vi "Delivery_boa.vi"() -> ()   [LabVIEW 2016]
uses:
  <vilib>/NXT/Subs/LVHSConnector.ctl
  <vilib>/NXT/LegoClasses/BrickReference/BrickReference.lvclass
  caracteristicas.ctl
  <vilib>/NXT/Subs/ColorSensorColors.ctl
  parametros.ctl
  <vilib>/NXT/Block Support/NXT_InputPort.ctl
  <vilib>/NXT/Block Support/NXT_OutputPort.ctl
  <vilib>/NXT/NXTIO Xnodes/NXTIONodeSubVIs/NXTMoveMotors.vi
  <vilib>/NXT/Dual Mode Library/Waits/Wait_Num.vi
  <vilib>/NXT/NXTIO Xnodes/NXTIONodeSubVIs/NXTStopMotors.vi
  <vilib>/NXT/NXTIO Xnodes/AddressXNode/NXTIOAddress.xnode
  <vilib>/NXT/NXTIO Xnodes/NXTIOXNode/NXTIO.xnode
panel:
  in  "Parâmetros Iniciais":T1={"Gyro Port"=0, "Sensor - Left"=3, "Sensor - Right"=2, "     Color \nSensor Port"=1, "Kp Front"=0.6, "Motor speed"=-15, "Distance to street"=20.0, "Motor speed turns"=16, "Kp Curvas"=0.3} {"Kp Front" format="%.3f"; "Color \nSensor Port" items=["Port 1", "Port 2", "Port 3", "Port 4"]; "Sensor - Right" items=["Port 1", "Port 2", "Port 3", "Port 4"]; "Sensor - Left" items=["Port 1", "Port 2", "Port 3", "Port 4"]; "Gyro Port" items=["Port 1", "Port 2", "Port 3", "Port 4"]}
  in  "Características Iniciais":T3={"Colors and Directions"=[enum."Zero", enum."Zero", enum."Zero", enum."Zero", enum."Zero", enum."Zero"], "Direction"=enum."Zero", "CS"=enum."Street", "Old Color"=enum."White"}
  out "Boolean":bool=TRUE
  in  "NXT/EV3":T5
  # "black"
  # "blue"
  # "green"
  # "yellow"
  # "red"
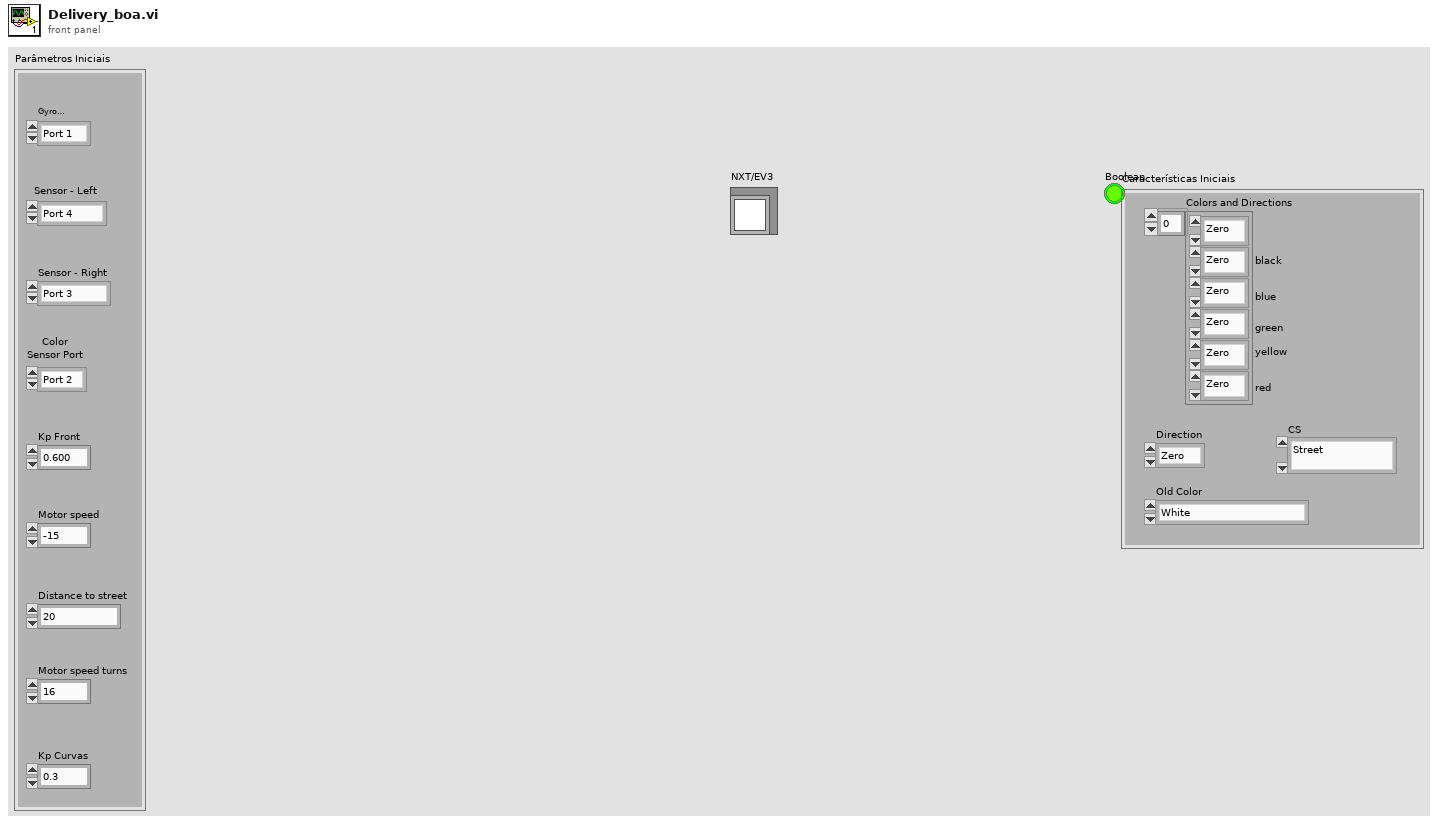
[diagram p1: front panel]
types:
  T1 = typedef "parametros.ctl" = cluster{"Gyro Port":T2, "Sensor - Left":T2, "Sensor - Right":T2, "     Color \nSensor Port":T2, "Kp Front":dbl, "Motor speed":i32, "Distance to street":dbl, "Motor speed turns":i32, "Kp Curvas":dbl}
  T2 = typedef "NXT_InputPort.ctl" = u32
  T3 = typedef "caracteristicas.ctl" = cluster{"Colors and Directions":enum16{"Zero", "Right", "Front", "Left"}[], "Direction":enum16{"Zero", "Right", "Front", "Left"}, "CS":enum16{"Street", "Intersection", "End", "Stop", "Square", "Delivery", "Empty"}, "Old Color":T4}
  T4 = typedef "ColorSensorColors.ctl" = enum16{"No Color", "Black", "Blue", "Green", "Yellow", "Red", "White", "Brown"}
  T5 = typedef "LVHSConnector.ctl" = refnum<class "BrickReference.lvclass">
  T6 = typedef "NXT_OutputPort.ctl" = u8
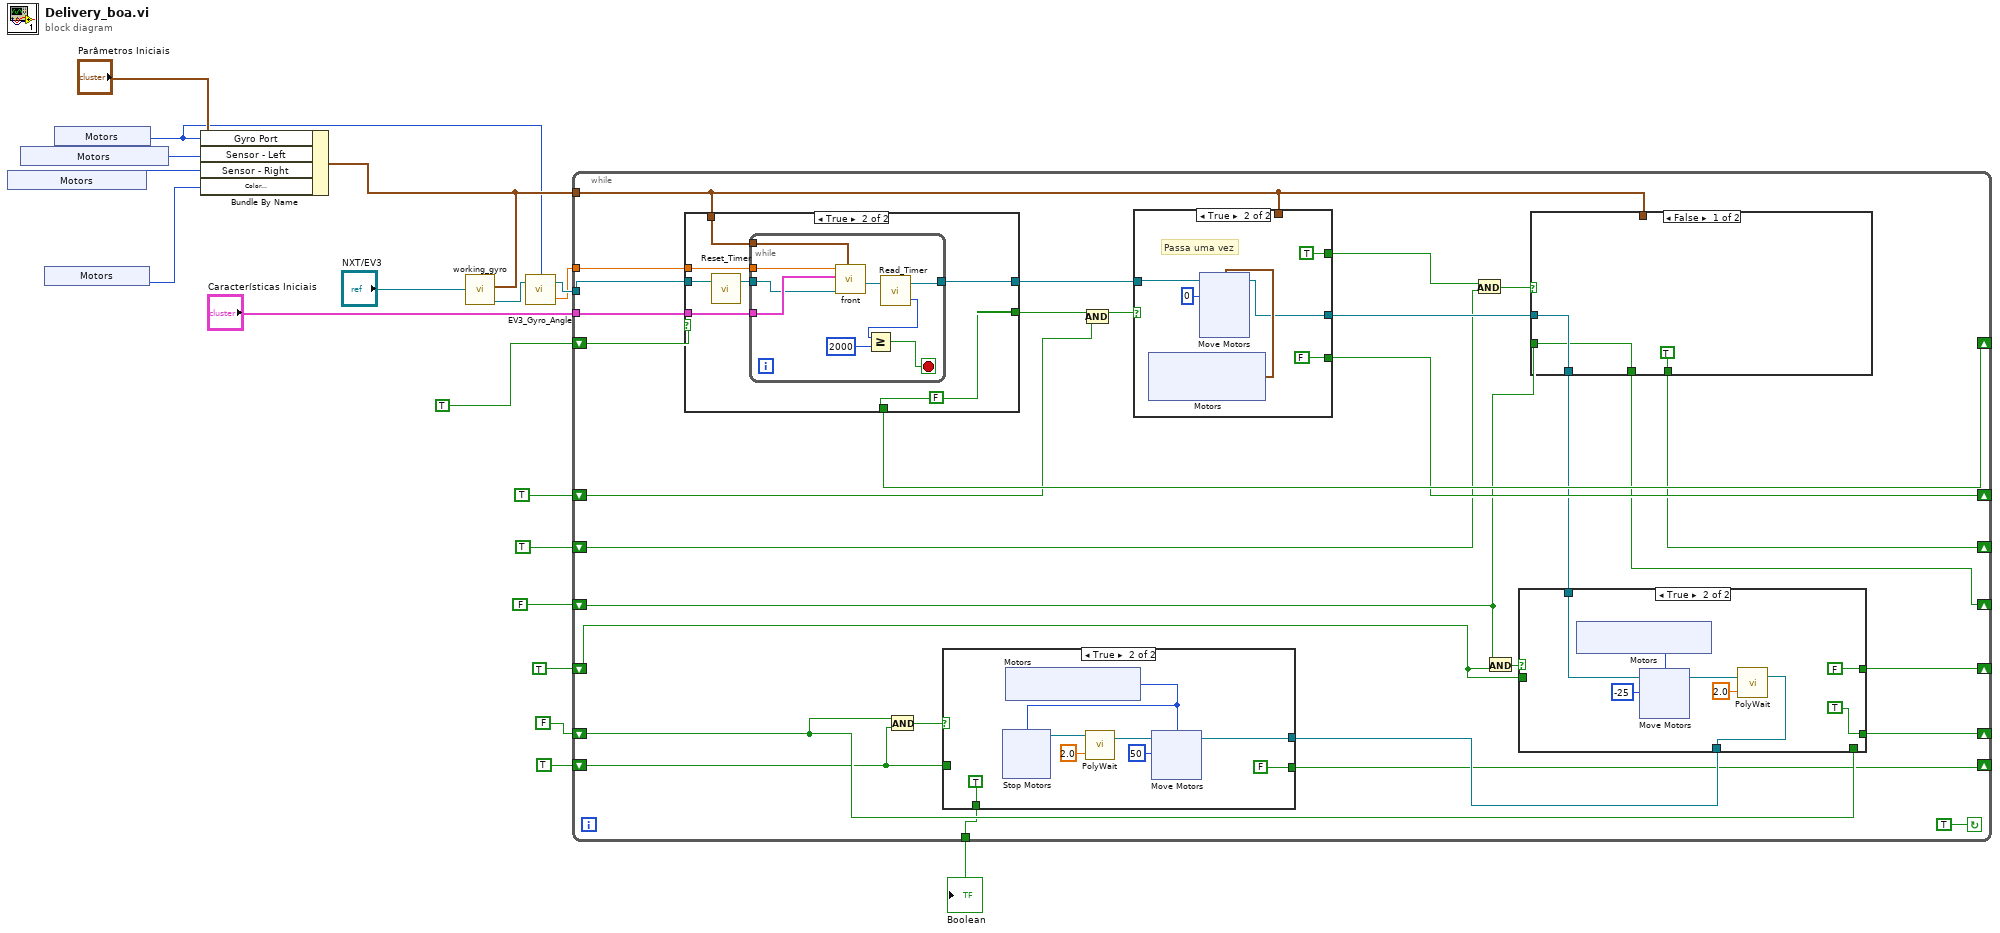
[diagram p0: block diagram]
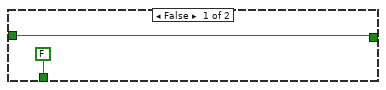
[diagram p2: hidden frame]
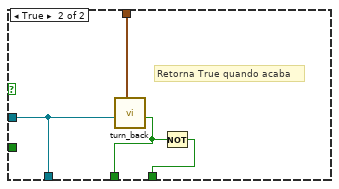
[diagram p4: hidden frame]
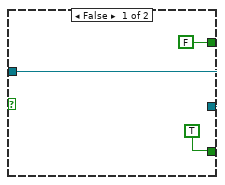
[diagram p5: hidden frame]
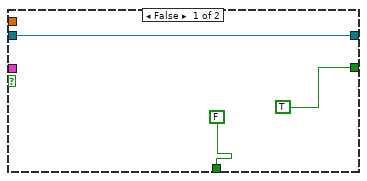
[diagram p6: hidden frame]
diagram:
  n1 = xnode "Motors"() -> ("Sensor"=w8:T2)
  n2 = xnode "Motors"() -> ("Sensor"=w9:T2)
  n3 = xnode "Motors"() -> ("Sensor"=w7:T2)
  n4 = xnode "Motors"() -> ("Sensor"=w1:T2)
  n5 = Bundle By Name(cluster="Parâmetros Iniciais", "Gyro Port"=w1, "Sensor - Left"=w9, "Sensor - Right"=w8, "Color \nSensor Port"=w7) -> (w5:T1)
  n6 = call "working_gyro.vi"("Parâmetros Iniciais"=w5, "NXT/EV3"="NXT/EV3") -> ("NXT/EV3 2"=w3:T5)  [unwired: 9 in]
  n7 = call <vilib>:"EV3_Gyro_Angle.vi"("NXT/EV3"=w3, "Port (Port 1)"=w1) -> ("Degrees"=w2:sgl, "NXT/EV3"=w4:T5)  [unwired: 1 in]
  n8 = while {
    tunnel: w4 -> [w49]
    tunnel: w2 -> [w48]
    shift-right: [w45] -> _
    shift-left: TRUE -> [w47]
    shift-right: [w40] -> _
    shift-left: TRUE -> [w43]
    tunnel: w5 -> [w20]
    shift-right: [w36] -> _
    shift-left: TRUE -> [w38]
    shift-right: [w34] -> _
    shift-left: FALSE -> [w32]
    shift-right: [w31] -> _
    shift-left: TRUE -> [w30]
    shift-right: [w28] -> _
    shift-left: FALSE -> [w26]
    shift-right: [w25] -> _
    shift-left: TRUE -> [w24]
    tunnel: [w23] -> w12
    tunnel: "Características Iniciais" -> [w21]
    stop <- TRUE continue-if-true
    n9 = case shown="True" w47 {
      tunnel: w49 -> [w118 w122]
      tunnel: w48 -> [_ w126]
      tunnel: [TRUE w125] -> w44
      tunnel: [w118 w120] -> w46
      tunnel: [FALSE w125] -> w45
      tunnel: w21 -> [_ w124]
      tunnel: w20 -> [_ w123]
      frame False {
      }
      frame True {
        w125 = FALSE
        n10 = call <vilib>:"Reset_Timer.vi"("NXT/EV3"=w122) -> ("NXT/EV3"=w121:T5)  [unwired: 3 in]
        n11 = while {
          tunnel: w126 -> [w135]
          tunnel: w124 -> [w134]
          tunnel: w123 -> [w133]
          tunnel: w121 -> [w132]
          tunnel: [w130] -> w120
          stop <- w127 stop-if-true
          n12 = call "front.vi"("Parâmetros Ini 2"=w133, "NXT/EV3"=w132, "Características Ini"=w134, "First Angle"=w135) -> ("NXT/EV3 2"=w131:T5)  [unwired: 7 in]
          n13 = call <vilib>:"Read_Timer.vi"("NXT/EV3"=w131) -> ("Value (msec)"=w129:u32, "NXT/EV3"=w130:T5)  [unwired: 2 in]
          n14 = Greater Or Equal?(x=w129, y=u32 2000) -> (x >= y?=w127:bool)
        }
      }
    }
    n15 = And(x=w26, y=w24) -> (x .and. y?=w27:bool)
    n16 = And(x=w44, y=w43) -> (x .and. y?=w42:bool)
    n17 = case shown="True" w42 {
      tunnel: w46 -> [w101 w105]
      tunnel: w20 -> [_ _]
      tunnel: [w101 w102] -> w41
      tunnel: [TRUE FALSE] -> w40
      tunnel: [FALSE TRUE] -> w37
      frame False {
      }
      frame True {
        w103 = i8 0 ("Power/Speed 1")
        # "Passa uma vez"
        n18 = xnode "Motors"() -> ("Motor"=w104:cluster{"Port":T6, "Port":T6})
        n19 = xnode "Move Motors"("Power/Speed 2"=w103, "Power/Speed 1"=w103, "Motors"=w104, "NXT/EV3"=w105) -> ("NXT/EV3"=w102:T5)
      }
    }
    n20 = And(x=w37, y=w38) -> (x .and. y?=w39:bool)
    n21 = And(x=w32, y=w30) -> (x .and. y?=w33:bool)
    n22 = case shown="False" w39 {
      tunnel: w41 -> [w93 w96]
      tunnel: [TRUE ("x = y?") w98] -> w36
      tunnel: w20 -> [_ w97]
      tunnel: [w93 w96] -> w35
      tunnel: [w92 w95] -> w34
      tunnel: w32 -> [w92 _]
      frame False {
      }
      frame True {
        # "Retorna True quando acaba"
        n23 = call "turn_back.vi"("Parâmetros Ini 2"=w97, "NXT/EV3"=w96) -> ("x = y?"=w95:bool)  [unwired: 8 in]
        n24 = Not(x=w95) -> (.not. x?=w98:bool)
      }
    }
    n25 = case shown="True" w33 {
      tunnel: w35 -> [w74 w81]
      tunnel: [w75 FALSE] -> w31
      tunnel: w30 -> [w75 _]
      tunnel: [w74 w77] -> w29
      tunnel: [w73 TRUE] -> w28
      tunnel: w26 -> [w73 _]
      frame False {
      }
      frame True {
        n26 = xnode "Motors"() -> ("Motor"=w83:T6)
        n27 = xnode "Move Motors"("Power/Speed 1"=i8 -25, "Motors"=w83, "NXT/EV3"=w81) -> ("NXT/EV3"=w78:T5)
        n28 = call-poly <vilib>:"PolyWait.vi"("Time (1 sec)"=sgl 2.0, "NXT/EV3"=w78) -> ("NXT/EV3"=w77:T5)  [unwired: 2 in]
      }
    }
    n29 = case shown="True" w27 {
      tunnel: w29 -> [_ w59]
      tunnel: [w51 FALSE] -> w25
      tunnel: w24 -> [w51 _]
      tunnel: [FALSE TRUE] -> w23
      frame False {
      }
      frame True {
        n30 = xnode "Motors"() -> ("Motor"=w54:T6)
        n31 = xnode "Move Motors"("Power/Speed 1"=i8 50, "Motors"=w54, "NXT/EV3"=w59) -> ("NXT/EV3"=w56:T5)
        n32 = call-poly <vilib>:"PolyWait.vi"("Time (1 sec)"=sgl 2.0, "NXT/EV3"=w56) -> ("NXT/EV3"=w55:T5)  [unwired: 2 in]
        n33 = xnode "Stop Motors"("Motors"=w54, "NXT/EV3"=w55) -> ()  [unwired: 1 out]
      }
    }
  }
  "Boolean" <- w12
